vi "Anti Elevator Death.vi"(0 "Motor Right":dbl, 1 "Motor Left":dbl, 3 "2nd Gear?":bool) -> (7 "Motor Right Output":dbl, 8 "Motor Left Output":dbl, 10 "2nd Gear?":bool)   [LabVIEW 2017]
uses:
  Robot Global Data.vi
  <vilib>/express/express arith-compare/Formula/XNode/ExpressFormulaBlockNode.xnode
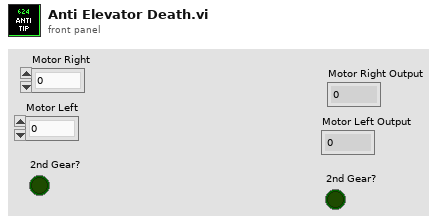
[diagram p1: front panel]
types:
  T1 = typedef "Dashboard Control Data.ctl" = cluster{"Drivetrain Settings Cluster":T2, "Intake Presets":T5, "Elevator Settings Cluster":T6, "Drivetrain Encoder Values":T8, "Auton Chooser":T9, "Auton Presets":cluster{"Start Position":dbl}, "Elevator Encoder Values":T10, "Pressure M":dbl, "Pressure B":dbl, "Zero All?":bool, "Enable Vision":bool}
  T2 = typedef "Drivetrain Settings Cluster.ctl" = cluster{"Gyro Steer PID Gains":T3, "Distance Drive PID Gains":T3, "Drive Tolerance":dbl, "Gyro Tolerance":dbl, "Gyro Output":dbl, "Distance Output":dbl, "Y Power Multiplier":dbl, "Turn Power Multiplier":dbl, "Creep Rate":dbl, "Encoder Reset":bool, "DT Mode Modifier":enum16{"None, Default", "Cube", "Square"}, "Left Encoder Tick Constant":dbl, "Right Encoder Tick Constant":dbl, "Shift Speed":dbl, "Zero Gyro":bool, "Y min":dbl, "Y max":dbl, "X min":dbl, "X max":dbl, "Finish Velocity":dbl, "Anti-Tip Settings":T4}
  T3 = typedef "PID Gains Cluster.ctl" = cluster{"Proportional Gain":dbl, "Integral Time":dbl, "Derivative Time":dbl}
  T4 = typedef "Anti-Tip Settings.ctl" = cluster{"Pitch Tip Constant":dbl, "Wheel Diameter":dbl, "Gearbox Reduction":dbl, "Motor Count":dbl, "Mass of Robot":dbl, "Almost Tip Constant":dbl, "Dist to CG":dbl}
  T5 = typedef "Intake Presets.ctl" = cluster{"Idle Angle":dbl, "Mid Angle":dbl, "Low Angle":dbl, "Outtake Power":dbl, "Intake Power":dbl, "Unstuck":dbl, "Angle Tolerance":dbl, "Max Angle":dbl, "Max Current":dbl, "Current Trip Time":dbl, "Reset Encoder?":bool, "Encoder Scale":dbl, "PID gains":cluster{"proportional gain (Kc)":dbl, "integral time (Ti, min)":dbl, "derivative time (Td, min)":dbl}, "output range":cluster{"output high":dbl, "output low":dbl}, "IR Constant Pull Rate":dbl, "Shoot Angle":dbl}
  T6 = typedef "Elevator Settings Cluster.ctl" = cluster{"Ground Height":dbl, "Switch Height":dbl, "Scale High Height ":dbl, "Scale Low Height":dbl, "Elevator PID Gains":T7, "Elevator Tolerance":dbl, "Reset Encoders":bool, "Encoder Scale":dbl, "Max Height":dbl, "Mid Height":dbl, "output range":cluster{"output high":dbl, "output low":dbl}, "Upper Slow Down Tolerance":dbl, "Tick Constant":dbl, "Tip Constant":dbl, "Slow Down Multiplier":dbl, "Almost Tip Constant":dbl, "Bottom Trip Offset":dbl, "Lower Slow Down Tolerance":dbl}
  T7 = typedef "PID Gains.ctl" = cluster{"proportional gain (Kc)":dbl, "integral time (Ti, min)":dbl, "derivative time (Td, min)":dbl}
  T8 = typedef "DT Encoder Values.ctl" = cluster{"Left Encoder":cluster{"Distance":dbl, "Speed":dbl, "Tick":dbl}, "Right Encoder":cluster{"Distance":dbl, "Speed":dbl, "Tick":dbl}}
  T9 = typedef "Auton Chooser.ctl" = cluster{"Left":bool, "Center":bool, "Right":bool, "Scale":bool, "Both":bool, "Switch":bool, "Test":bool, "No Script":bool, "Drive PID":bool, "Elevator PID":bool, "Gyro PID":bool}
  T10 = typedef "Elevator Encoder Values.ctl" = cluster{"Encoder Values":cluster{"Distance":dbl, "Speed":dbl, "Tick":dbl}}
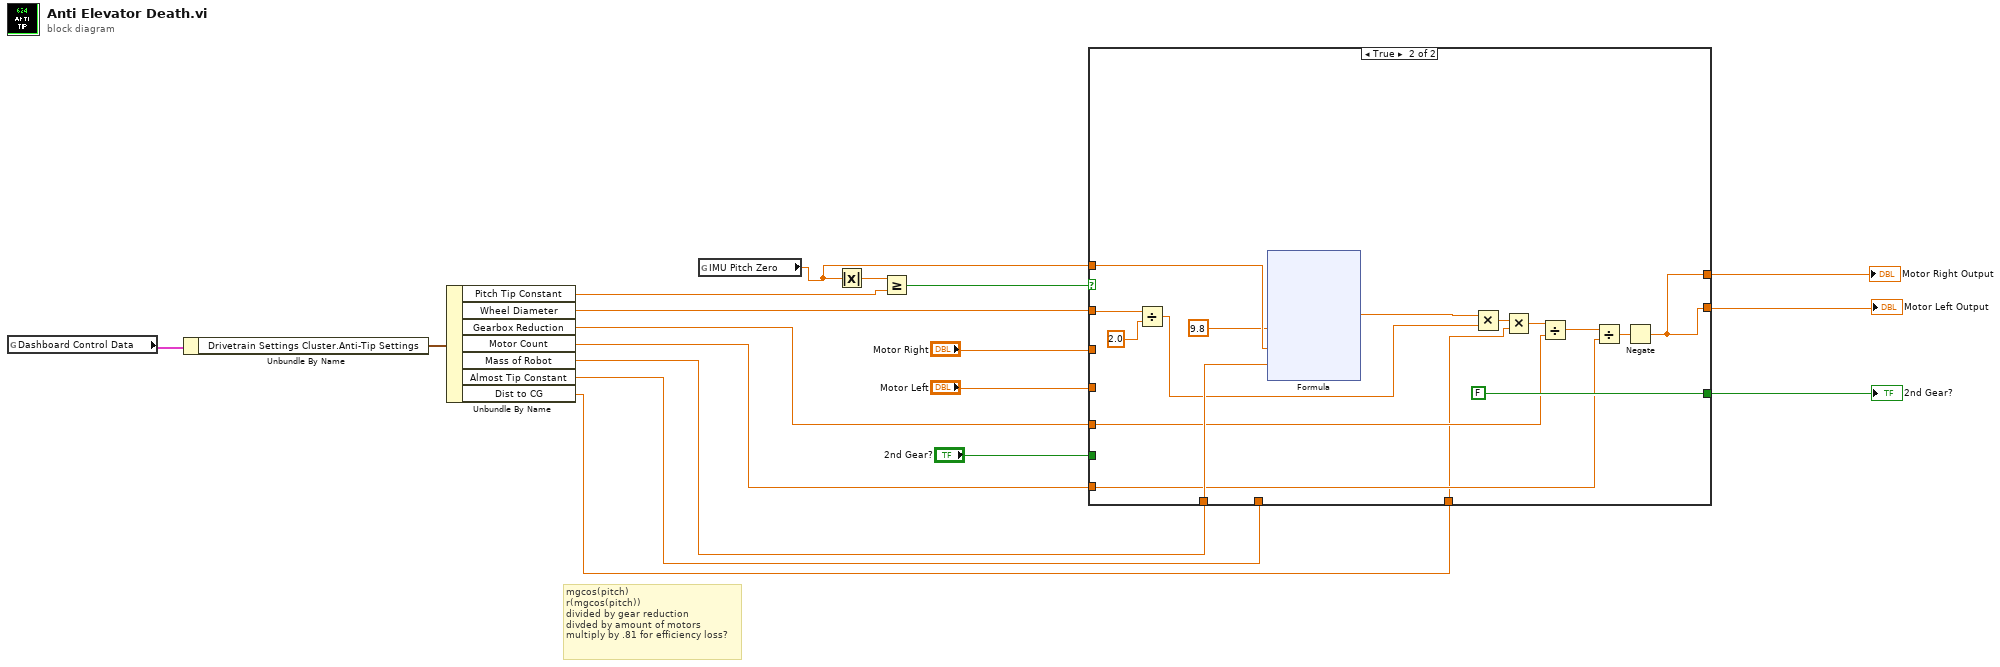
[diagram p0: block diagram]
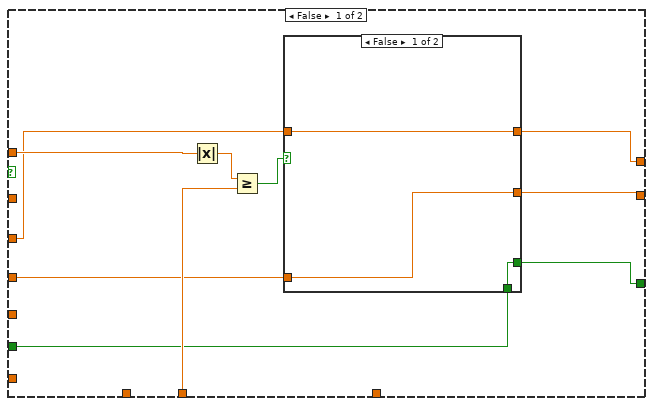
[diagram p2: hidden frame]
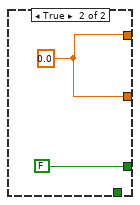
[diagram p3: hidden frame]
diagram:
  # "mgcos(pitch)\nr(mgcos(pitch))\ndivided by gear reduction\ndivded by amount of motors\nmultiply by .81 for efficiency loss?"
  n1 = global read "Robot Global Data.vi" "Dashboard Control Data"() -> (w18:T1)
  n2 = Unbundle By Name(w18) -> ("Drivetrain Settings Cluster.Anti-Tip Settings"=w8:T4)
  n3 = Unbundle By Name(w8) -> ("Pitch Tip Constant"=w7:dbl, "Wheel Diameter"=w6:dbl, "Gearbox Reduction"=w5:dbl, "Motor Count"=w4:dbl, "Mass of Robot"=w3:dbl, "Almost Tip Constant"=w2:dbl, "Dist to CG"=w1:dbl)
  n4 = global read "Robot Global Data.vi" "IMU Pitch Zero"() -> (w16:dbl)
  n5 = Absolute Value(x=w16) -> (abs(x)=w15:dbl)
  n6 = Greater Or Equal?(x=w15, y=w7) -> (x >= y?=w17:bool)
  n7 = case shown="True" w17 {
    tunnel: w16 -> [w28 w47]
    tunnel: [w22 w34] -> w14
    tunnel: [w23 w34] -> w13
    tunnel: [w24 FALSE] -> w12
    tunnel: "Motor Right" -> [w21 _]
    tunnel: "Motor Left" -> [w20 _]
    tunnel: "2nd Gear?" -> [w19 _]
    tunnel: w6 -> [_ w44]
    tunnel: w5 -> [_ w41]
    tunnel: w4 -> [_ w39]
    tunnel: w3 -> [_ w48]
    tunnel: w2 -> [w26 _]
    tunnel: w1 -> [_ w36]
    frame False {
      n8 = Absolute Value(x=w28) -> (abs(x)=w27:dbl)
      n9 = Greater Or Equal?(x=w27, y=w26) -> (x >= y?=w25:bool)
      n10 = case shown="False" w25 {
        tunnel: [w31 w33] -> w22
        tunnel: [w30 w33] -> w23
        tunnel: [w29 FALSE] -> w24
        tunnel: w21 -> [w31 _]
        tunnel: w20 -> [w30 _]
        tunnel: w19 -> [w29 _]
        frame False {
        }
        frame True {
          w33 = 0.0
        }
      }
    }
    frame True {
      n11 = Divide(x=w44, y=2.0) -> (x/y=w42:dbl)
      n12 = xnode "Formula"("Gravitational Constant"=9.8, "Pitch"=w47, "Mass"=w48) -> ("Result"=w45:dbl)  [unwired: 1 in, 1 out]
      n13 = Multiply(x=w45, y=w42) -> (x*y=w38:dbl)
      n14 = Multiply(x=w38, y=w36) -> (x*y=w37:dbl)
      n15 = Divide(x=w37, y=w41) -> (x/y=w40:dbl)
      n16 = Divide(x=w40, y=w39) -> (x/y=w35:dbl)
      n17 = Negate(x=w35) -> (-x=w34:dbl)
    }
  }
  "Motor Right Output" <- w14
  "Motor Left Output" <- w13
  "2nd Gear?" <- w12
